vi "WS_RS485ETH_set.vi"(5 "param_num":string="1", 7 "address":string="022", 8 "error in":errorcluster, 9 "data":string="1", 10 "data_length":string="1", 11 "conn_id_in":refnum<k5>) -> (0 "error out":errorcluster, 1 "status":bool, 3 "conn_id_out":refnum<k5>)   [LabVIEW 2019]
panel:
  out "command":string
  in  "action":string="1"
  # "0 = data request, 1 = control command"
  # "3 digits"
  # "3 digits"
  # "2 digits"
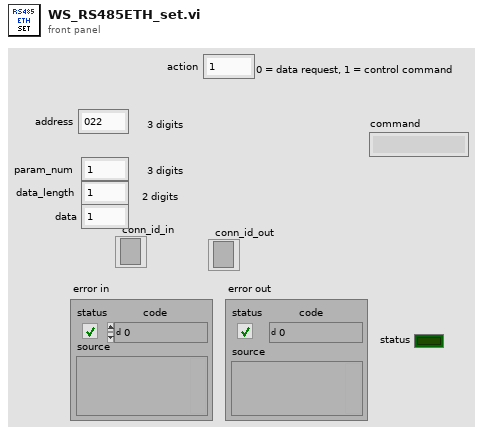
[diagram p1: front panel]
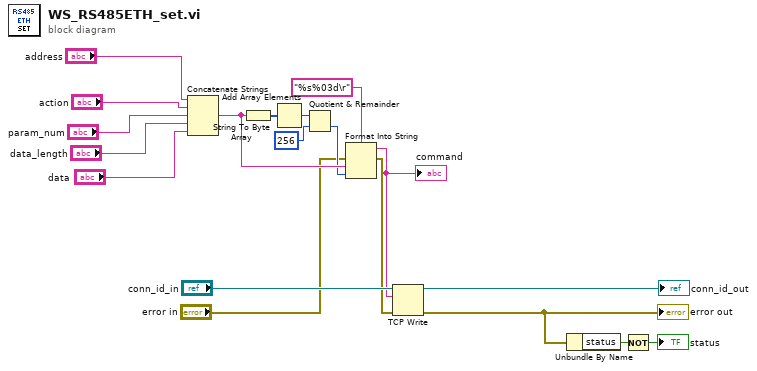
[diagram p0: block diagram]
diagram:
  n1 = Concatenate Strings("address", "action", "param_num", "data_length", "data") -> (w5:string)
  n2 = String To Byte Array(string=w5) -> (unsigned byte array=w9:u8[])
  n3 = Add Array Elements(numeric array=w9) -> (sum=w7:u8)
  n4 = Quotient & Remainder(x=w7, y=u64 256) -> (floor(x/y)=w4:u64)  [unwired: 1 out]
  n5 = Format Into String(format string="%s%03d\r", error in="error in", w5, w4) -> (resulting string=w3:string, error out=w1:errorcluster)  [unwired: 1 in]
  "command" <- w3
  n6 = TCP Write(connection ID="conn_id_in", data in=w3, error in (no error)=w1) -> (connection ID out=→"conn_id_out":refnum<k5>, error out=w19:errorcluster)  [unwired: 1 in, 1 out]
  "error out" <- w19
  n7 = Unbundle By Name(w19) -> ("status"=w16:bool)
  n8 = Not(x=w16) -> (.not. x?=→"status":bool)
